vi "test_Move Slot.vi"(8 "error in (no error)":errorcluster, 11 "TestCase in":refnum<class "Scan Engine Scripting API Custom Device Unit Tests.lvclass">) -> (0 "error out":errorcluster, 3 "TestCase out":refnum<class "Scan Engine Scripting API Custom Device Unit Tests.lvclass">)   [LabVIEW 2017, in "Scan Engine Scripting API Custom Device Unit Tests.lvclass"]
uses:
  Scan Engine Scripting API Custom Device Unit Tests.lvclass
  Type Defs/Local Chassis Settings.ctl
  Scripting/Modules/Module/Module.lvclass
  Scripting/Modules/Mode Classes/Counter Driven Output Mode/Drive from Slot.ctl
  Scripting/Modules/NI 9474/NI 9474.lvclass
  C:/dev/niveristand-scan-engine-ethercat-custom-device/Custom Device Source/Scripting/Modules/Module/Module.lvclass
  Scan Engine Scripting API Custom Device Unit Tests.lvclass/Scan Engine Scripting API Custom Device Unit Tests.ctl
  Type Defs/Main Settings.ctl
  c7e83f66-a965-41fd-b07a-d8c29414f51e.vi
  a134009e-d5c9-407c-b835-1c4aa24009a3.vi
  Utility/Set Error.vi
  <vilib>/Utility/error.llb/Clear Errors.vi
  Modules.lvlibp/SD Module/SD Module.lvclass
  C:/dev/niveristand-scan-engine-ethercat-custom-device/Custom Device Source/Modules.lvlibp/RSI Module/RSI Module.lvclass
  Scripting/Modules/NI 9224/NI 9224.lvclass
  Scripting/Modules/NI 9228/NI 9228.lvclass
  Modules.lvlibp/RSI Module/Read Module Page Property.vi
  Modules.lvlibp/RSI Module/Read Model.vi
  Scripting/Utility/Convert Module Model to Module Class.vi
  Modules.lvlibp/SD Module/Read DIO mode.vi
  Modules.lvlibp/RSI Module/Read Channels.vi
  Scripting/Utility/Convert to DI Module.vi
  Scripting/Utility/Convert to DO Module.vi
  Scripting/Utility/Convert to CI PWM Module.vi
  Scripting/Utility/Convert to CDO Module.vi
  Scripting/Utility/Convert to PWM Module.vi
  Globals/Error Strings.vi
  Scripting/Utility/Convert to AI Vrms Module.vi
  Scripting/Utility/Convert to AI Module.vi
  Modules.lvlibp/9224/9224.lvclass
  <vilib>/addons/_JKI Toolkits/VI Tester/TestCase.llb/TestCase.lvclass
  Scripting/Scan Engine Scripting.lvlib
  Scan Engine Custom Device.lvlib
  Scripting/Modules/Mode Classes/Counter Driven Output Mode/Counter Driven Output Mode.lvclass
  C:/Program Files (x86)/National Instruments/LabVIEW 2017/vi.lib/addons/_JKI Toolkits/VI Tester/TestCase.llb/TestCase.lvclass
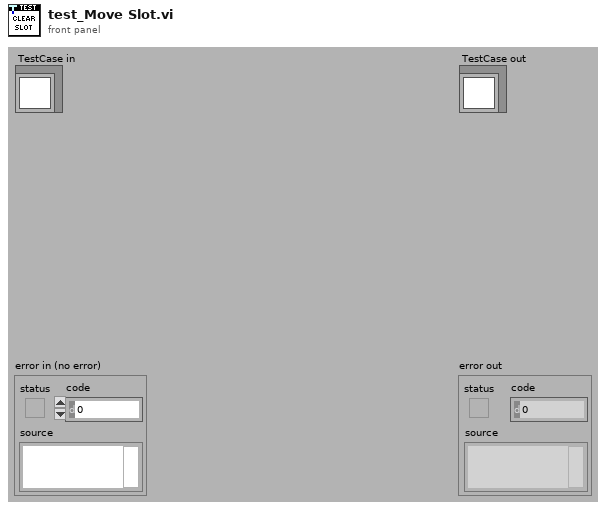
[diagram p1: front panel]
types:
  T1 = typedef "Scan Engine Scripting.lvlib/Counter Driven Output Mode.lvclass/Drive from Slot.ctl" = enum16{"Slot 1", "Slot 2", "Slot 3", "Slot 4", "Slot 5", "Slot 6", "Slot 7", "Slot 8"}
  T2 = typedef "Scan Engine Custom Device.lvlib/Local Chassis Settings.ctl" = cluster{"name":string, "number of slots":i32}
  T3 = typedef "Scan Engine Custom Device.lvlib/Main Settings.ctl" = cluster{"sync to scan":bool, "scan engine decimation":u16, "delay after FPGA load (s)":u16}
  T4 = typedef "Custom Device API.lvlib/Custom Device Item Ref.ctl" = u64
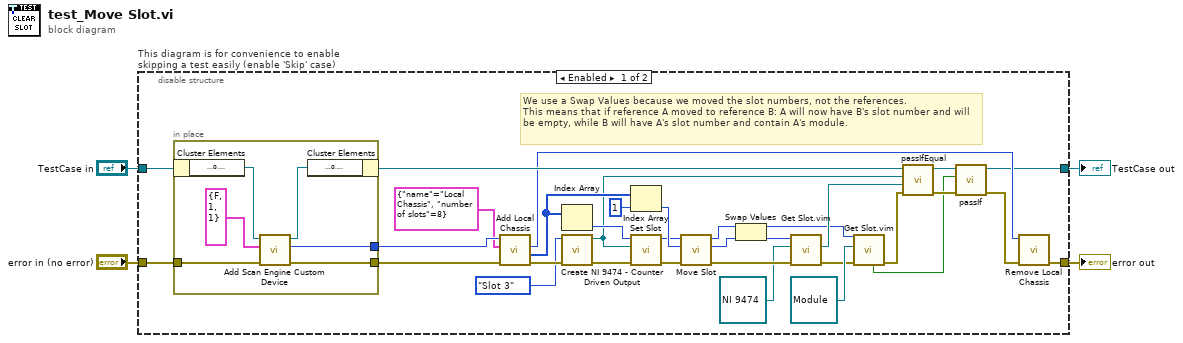
[diagram p0: block diagram]
diagram:
  n1 = disable-structure "This diagram is for convenience to enable skipping a test easily (enable 'Skip' case)" shown="Enabled" {
    disable-tunnel: "TestCase in" -> [w34 w47]
    disable-tunnel: [w14 w45] -> w1
    disable-tunnel: [w21 w46] -> w3
    disable-tunnel: "error in (no error)" -> [w35 w44]
    frame Enabled {
      # "We use a Swap Values because we moved the slot numbers, not the references.\nThis means that if reference A moved to reference B: A will now have B's slot number and will be empty, while B will have A's slot number and contain A's module."
      n2 = in-place {
        in-place-border: [w43] -> w37
        in-place-border: [w42] -> w36
        in-place-border: w35 -> [w40]
        n3 = in-place-cluster #1(w34) -> ("target ref"=w39:refnum<k24>)
        n4 = call "Add Scan Engine Custom Device.vi"("error in"=w40, "settings"=T3 {"sync to scan"=FALSE, "scan engine decimation"=1, "delay after FPGA load (s)"=1}, "target in"=w39) -> ("error out"=w42:errorcluster, "scan engine custom device ref"=w43:T4, "target out"=w38:refnum<k24>)  [unwired: 6 in]
        n5 = in-place-cluster #1("target ref"=w38) -> (w33:refnum<class "Scan Engine Scripting API Custom Device Unit Tests.lvclass">)
      }
      n6 = call "Add Local Chassis.vi"("error in"=w36, "settings"=T2 {"name"="Local Chassis", "number of slots"=8}, "scan engine custom device ref in"=w37) -> ("error out"=w30:errorcluster, "slot refs"=w27:T4[], "local chassis ref"=w32:T4)  [unwired: 4 in, 2 out]
      n7 = Index Array(array=w27) -> (element=w26:T4)  [unwired: 1 in]
      n8 = call "Create NI 9474 - Counter Driven Output.vi"("error in"=w30, "drive from slot"=Drive_from_Slot."Slot 3") -> ("error out"=w29:errorcluster, "NI 9474 out"=w17:refnum<class "NI 9474.lvclass">)  [unwired: 8 in]
      n9 = Index Array(array=w27, index=1) -> (element=w25:T4)
      n10 = call "Set Slot.vi"("error in"=w29, "module"=w17, "slot ref in"=w26) -> ("error out"=w31:errorcluster, "slot ref out"=w12:T4)  [unwired: 7 in]
      n11 = call "Move Slot.vi"("error in"=w31, "destination slot ref in"=w25, "source slot ref in"=w12) -> ("error out"=w24:errorcluster, "destination slot ref out"=w9:T4, "source slot ref out"=w10:T4)  [unwired: 6 in]
      n12 = Swap Values(12:w10, 14:w9) -> (1:w8:T4, 3:w7:T4)  [unwired: 1 in]
      n13 = call "Get Slot.vim"("error in"=w24, "module in"=refnum<class "NI 9474.lvclass"> refnum ("NI 9474 out"), "slot ref in"=w7) -> ("error out"=w22:errorcluster, "module"=w18:refnum<class "NI 9474.lvclass">)  [unwired: 5 in, 2 out]
      n14 = call "Get Slot.vim"("error in"=w22, "module in"=refnum<class "Module.lvclass"> refnum ("Scan Engine Scripting.lvlib:Module.lvclass"), "slot ref in"=w8) -> ("error out"=w19:errorcluster, "empty"=w13:bool)  [unwired: 5 in, 2 out]
      n15 = call-dynamic "passIfEqual.vi"("error in (no error)"=w19, "y"=w18, "x"=w17, "TestCase in"=w33) -> ("error out"=w20:errorcluster, "TestCase out"=w15:refnum<class "Scan Engine Scripting API Custom Device Unit Tests.lvclass">)  [unwired: 6 in]
      n16 = call-dynamic "passIf.vi"("error in (no error)"=w20, "pass"=w13, "TestCase in"=w15) -> ("error out"=w16:errorcluster, "TestCase out"=w14:refnum<class "Scan Engine Scripting API Custom Device Unit Tests.lvclass">)  [unwired: 7 in]
      n17 = call "Remove Local Chassis.vi"("error in"=w16, "local chassis ref"=w32) -> ("error out"=w21:errorcluster)  [unwired: 9 in]
    }
    frame Disabled {
      # "skip test result while test is under development"
      n18 = call <vilib>:"skip.vi"("error in (no error)"=w44, "TestCase in"=w47) -> ("error out"=w46:errorcluster, "TestCase out"=w45:refnum<class "Scan Engine Scripting API Custom Device Unit Tests.lvclass">)  [unwired: 8 in]
    }
  }
  "error out" <- w3
  "TestCase out" <- w1
